vi "Scan2graph.vi"() -> ()   [LabVIEW 2013]
panel:
  in  "Fit polynomiales":bool
  in  "Line Style":string(combo)="-"
  in  "Marker Shape":string(combo)="*"
  out "error out":errorcluster
  in  "Lancer Matlab":bool
  out "ListofColors":u32[](array[colorbox])
  in  "Array":i32[](array[numeric])
  out "OS":string
  in  "Polydegree Line Width":i32=2 min=0 max=15 step=1
  in  "PolyDegree":i32=3 min=0 max=69 step=1
  in  "Marker Size":i32=2 min=1 max=15 step=1
  in  "Line Width":i32=1 min=0 max=15 step=1
  in  "Wait":i32=3 min=0 max=15 step=1
  out "Nombre de couleur":i32
  out "Hauteur":i16
  out "Largeur":i16
  out "Image ˆ retravailler":picture
  in  "Selectionner une image *.png":path
  out "Affichage des erreurs":string
  # "ScanTest: panneau de control"
  # "Options du Graphique"
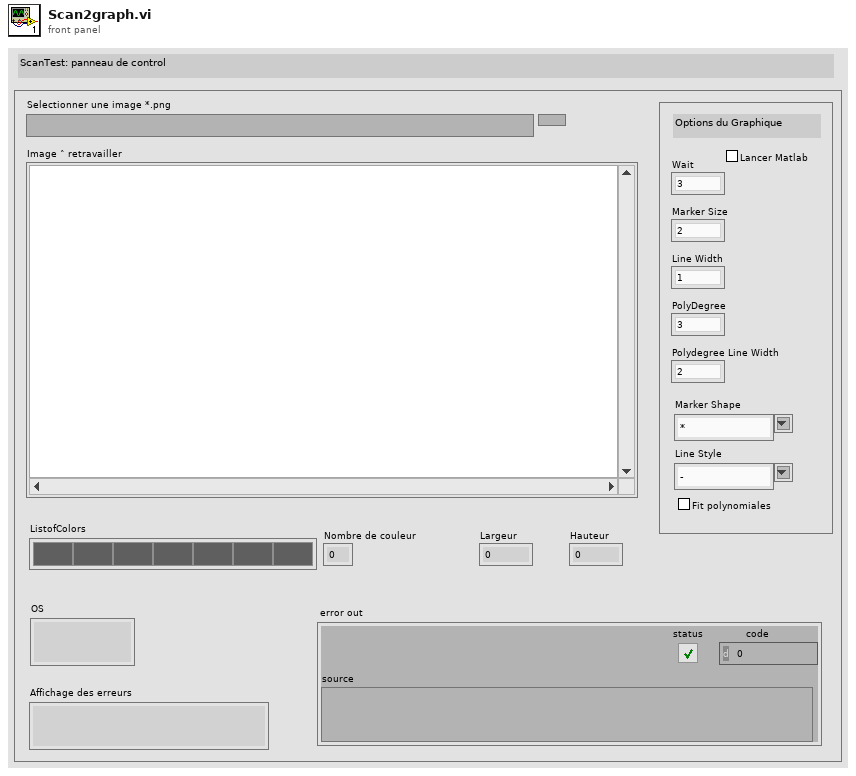
[diagram p1: front panel]
types:
  T1 = enum16{"open", "replace", "create", "open or create", "replace or create", "replace or create with confirmation"}
  T2 = typedef "imagedata.ctl" = cluster{"image type":i32, "image depth":i32, "image":u8[], "mask":u8[], "colors":u32[], "Rectangle":cluster{"left":i16, "top":i16, "right":i16, "bottom":i16}}
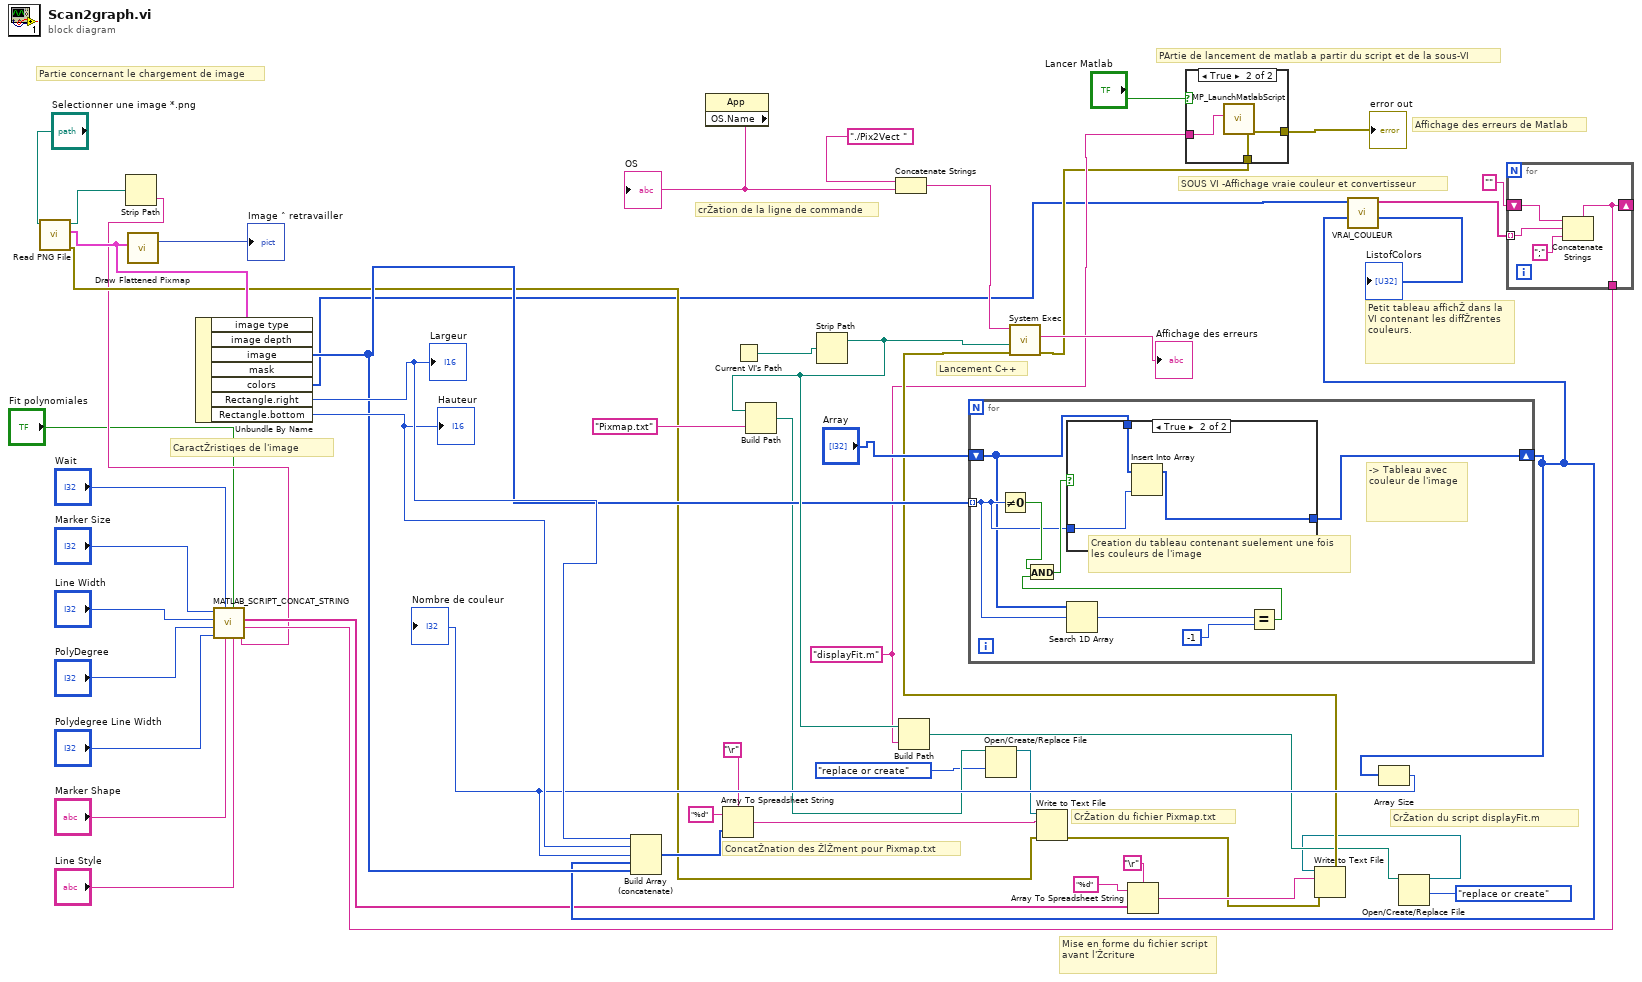
[diagram p0: block diagram]
diagram:
  w22 = "displayFit.m" ("name or relative path")
  # "crŽation de la ligne de commande"
  # "ConcatŽnation des ŽlŽment pour Pixmap.txt"
  # "CrŽation du fichier Pixmap.txt"
  # "Mise en forme du fichier script avant l'Žcriture"
  # "CrŽation du script displayFit.m"
  # "Petit tableau affichŽ dans la VI contenant les diffŽrentes couleurs."
  # "Lancement C++"
  # "Affichage des erreurs de Matlab"
  # "SOUS VI -Affichage vraie couleur et convertisseur"
  # "PArtie de lancement de matlab a partir du script et de la sous-VI"
  # "CaractŽristiqes de l'image"
  # "Partie concernant le chargement de image"
  n1 = call <vilib>:"Read PNG File.vi"("path to PNG file"="Selectionner une image *.png") -> ("error out"=w31:errorcluster, "image data"=w47:T2, "path"=w35:path)  [unwired: 8 in]
  n2 = Strip Path(path=w35) -> (name=w6:string)  [unwired: 1 out]
  n3 = call <vilib>:"Draw Flattened Pixmap.vi"("image data"=w47) -> ("new picture"=→"Image ˆ retravailler":picture)  [unwired: 8 in]
  n4 = Unbundle By Name(w47) -> ("image"=w33:u8[], "colors"=w17:u32[], "Rectangle.right"=w46:i16, "Rectangle.bottom"=w45:i16)  [unwired: 3 out]
  "Largeur" <- w46
  "Hauteur" <- w45
  n5 = property class="App"() -> ("OS.Name"=w21:string)  [unwired: 2 in, 2 out]
  "OS" <- w21
  n6 = Current VI's Path() -> (path=w51:path)
  n7 = Strip Path(path=w51) -> (stripped path=w36:path)  [unwired: 1 out]
  n8 = Build Path(base path=w36, name or relative path="Pixmap.txt") -> (appended path=w25:path)
  n9 = Concatenate Strings("./Pix2Vect ", w21) -> (w50:string)
  n10 = Build Path(base path=w36, name or relative path=w22) -> (appended path=w27:path)
  n11 = for {
    shift-right: [w57] -> w16
    shift-left: "Array" -> [w56]
    tunnel: w33 -> [w58] mode=indexing
    # "Creation du tableau contenant suelement une fois les couleurs de l'image"
    # "-> Tableau avec couleur de l'image"
    n12 = Not Equal To 0?(x=w58) -> (x != 0?=w60:bool)
    n13 = Search 1D Array(1D array=w56, element=w58) -> (index of element=w55:i32)  [unwired: 1 in]
    n14 = Equal?(x=w55, y=-1) -> (x = y?=w53:bool)
    n15 = And(x=w60, y=w53) -> (x .and. y?=w59:bool)
    n16 = case shown="True" w59 {
      tunnel: w56 -> [w61 w64]
      tunnel: [w61 w63] -> w57
      tunnel: w58 -> [_ w62]
      frame False {
      }
      frame True {
        n17 = Insert Into Array(array=w64, new element=w62) -> (w63:i32[])  [unwired: 1 in]
      }
    }
  }
  n18 = Open/Create/Replace File(file path (use dialog)=w25, operation (0:open)=T1."replace or create") -> (refnum out=w24:refnum<file>)  [unwired: 4 in, 2 out]
  n19 = call "VRAI_COULEUR.vi"("IMAGE COLORS"=w16, "CLUT"=w17) -> ("REAL IMAGE COLORS"=→"ListofColors":i32[], "STRING FOR MATLAB"=w15:string[])  [unwired: 8 in]
  n20 = Array Size(array=w16) -> (size(s)=w43:i32)
  "Nombre de couleur" <- w43
  n21 = Build Array (concatenate)(w46, w45, w43, w16, w33) -> (w44:i32[])
  n22 = Array To Spreadsheet String(delimiter (Tab)="\r", array=w44, 3:"%d" ("format string")) -> (spreadsheet string=w40:string)
  n23 = Write to Text File(file (use dialog)=w24, text=w40, error in=w31) -> (error out=w30:errorcluster)  [unwired: 1 in, 2 out]
  n24 = Open/Create/Replace File(file path (use dialog)=w27, operation (0:open)=T1."replace or create") -> (refnum out=w26:refnum<file>)  [unwired: 4 in, 2 out]
  n25 = for {
    shift-right: [w67] -> _
    shift-left: "" -> [w68]
    tunnel: w15 -> [w66] mode=indexing
    tunnel: [w67] -> w13
    n26 = Concatenate Strings(w68, w66, ";" ("string")) -> (w67:string)
  }
  n27 = call "MATLAB_SCRIPT_CONCAT_STRING.vi"("FILENAME"=w6, "COLOR_STR"=w13, "Line Style"="Line Style", "Fit polynomiales"="Fit polynomiales", "Marker Shape"="Marker Shape", "Wait"="Wait", "Polydegree Line Width"="Polydegree Line Width", "PolyDegree"="PolyDegree", "Line Width"="Line Width", "Marker Size"="Marker Size") -> ("SCRIPT_STR"=w12:string[])  [unwired: 1 in]
  n28 = Array To Spreadsheet String(delimiter (Tab)="\r", array=w12, 3:"%d" ("format string")) -> (spreadsheet string=w37:string)
  n29 = Write to Text File(file (use dialog)=w26, text=w37, error in=w30) -> (error out=w29:errorcluster)  [unwired: 1 in, 2 out]
  n30 = call <vilib>:"System Exec.vi"("error in (no error)"=w29, "working directory"=w36, "command line"=w50) -> ("error out"=w20:errorcluster, "standard error"=→"Affichage des erreurs":string)  [unwired: 5 in, 2 out]
  n31 = case shown="True" "Lancer Matlab" {
    tunnel: w22 -> [_ w72]
    tunnel: w20 -> [w69 w71]
    tunnel: [w69 w70] -> w19
    frame False {
    }
    frame True {
      n32 = call "MP_LaunchMatlabScript.vi"("error in (no error)"=w71, "matlab script name with extension"=w72) -> ("error out"=w70:errorcluster)  [unwired: 5 in, 4 out]
    }
  }
  "error out" <- w19
